vi "Load Config.vi"(8 "error in (no error)":errorcluster, 11 "DigitalInChannel in":refnum<class "DigitalInChannel.lvclass">) -> (0 "error out":errorcluster, 3 "DigitalInChannel out":refnum<class "DigitalInChannel.lvclass">)   [LabVIEW 2020, in "VolatusDAQConfig.lvlib" / "DigitalInChannel.lvclass"]
uses:
  DigitalInChannel.lvclass
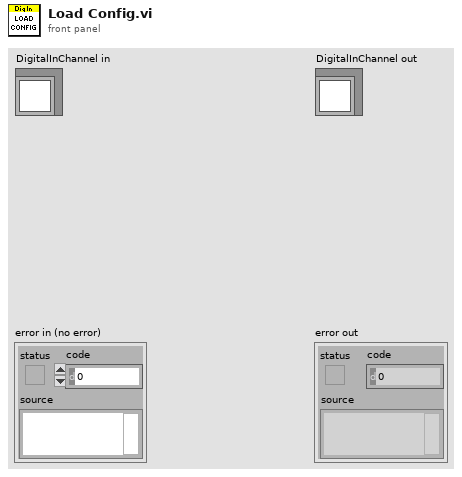
[diagram p1: front panel]
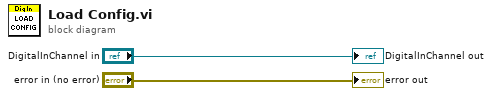
[diagram p0: block diagram]
diagram:
  "error out" <- "error in (no error)"
  "DigitalInChannel out" <- "DigitalInChannel in"
